vi "WFCompose.vi"   [LabVIEW 2013]
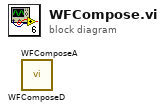
[diagram p0: block diagram]
diagram:
  n1 = call "WFComposeD.vi"() -> ()  [unwired: 10 in, 2 out]
  n2 = call "WFComposeA.vi"() -> ()  [unwired: 10 in, 2 out]
